vi "Write Loop Structure.vi"(8 "error in (no error)":errorcluster, 10 "Loop Structure":refnum<vi>, 11 "Module Loop in":refnum<class "Module Loop.lvclass">) -> (0 "error out":errorcluster, 3 "Module Loop out":refnum<class "Module Loop.lvclass">)   [LabVIEW 2015, in "Module Loop.lvclass"]
uses:
  Module Loop.lvclass
  Module Loop.lvclass/Module Loop.ctl
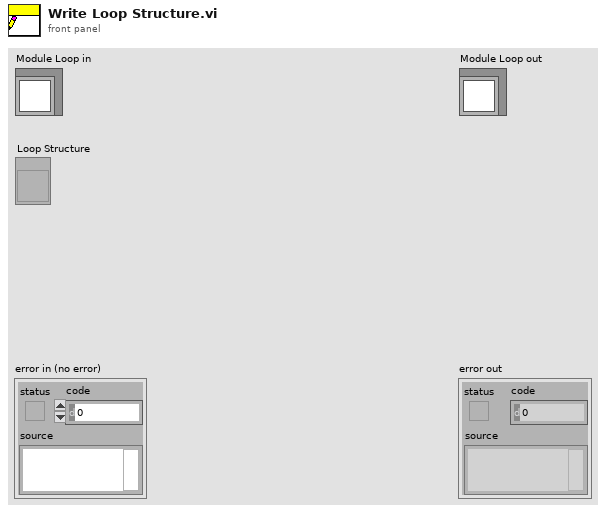
[diagram p1: front panel]
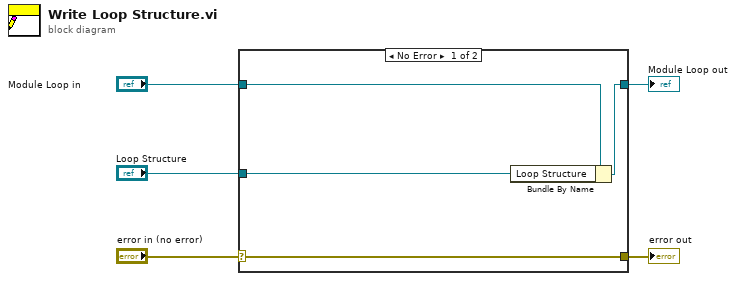
[diagram p0: block diagram]
diagram:
  n1 = case shown="No Error" "error in (no error)" {
    selector: "error in (no error)" -> [w9 w10]
    tunnel: [w9 w10] -> w4
    tunnel: [w7 w11] -> w2
    tunnel: "Module Loop in" -> [w8 w11]
    tunnel: "Loop Structure" -> [w6 _]
    frame No Error {
      n2 = Bundle By Name(cluster=w8, "Loop Structure"=w6) -> (w7:refnum<class "Module Loop.lvclass">)
    }
    frame Error {
    }
  }
  "error out" <- w4
  "Module Loop out" <- w2
